vi "myRIO v1.0 Generate Register Values SPI.vi"(8 "error in (no error)":errorcluster, 11 "SPI Configuration v1.0":T1={"Frequency (Hz)"=0.0, "SPI Clock Phase"=enum."Leading", "SPI Clock Polarity"=enum."Low", "SPI Data Direction"=enum."Most significant bit first", "Frame Length"=1} {"Frame Length" min=1 max=16}) -> (0 "error out":errorcluster, 2 "SPI.CNFG":u16 format="%.0b", 3 "SPI.CNT":u16, 5 "Actual Frequency (Hz)":dbl)   [LabVIEW 2021]
uses:
  <vilib>/myRIO/Common/Instrument Driver Framework/myRIO v1.0/SPI/typedefs/SPI Configuration v1.0.ctl
  <vilib>/myRIO/Common/Instrument Driver Framework/myRIO v1.0/SPI/typedefs/SPI Clock Phase.ctl
  <vilib>/myRIO/Common/Instrument Driver Framework/myRIO v1.0/SPI/typedefs/SPI Clock Polarity.ctl
  <vilib>/myRIO/Common/Instrument Driver Framework/myRIO v1.0/SPI/typedefs/SPI Data Direction.ctl
  <vilib>/myRIO/Common/Instrument Driver Framework/myRIO v1.0/SPI/typedefs/SPI Frame Length.ctl
  <vilib>/myRIO/Common/Instrument Driver Framework/Utilities/typedefs/Clock Calculation Parameters.ctl
  <vilib>/myRIO/Common/Instrument Driver Framework/Utilities/vis/Calculate TOP (Phase Correct Mode).vi
  <vilib>/myRIO/Common/Instrument Driver Framework/Utilities/vis/Calculate TOP (Normal Mode).vi
  <vilib>/myRIO/Common/Instrument Driver Framework/Utilities/vis/Calculate Frequency (Phase Correct Mode).vi
  <vilib>/myRIO/Common/Instrument Driver Framework/Utilities/vis/Calculate Frequency (Normal Mode).vi
  <vilib>/Utility/error.llb/Error Cluster From Error Code.vi
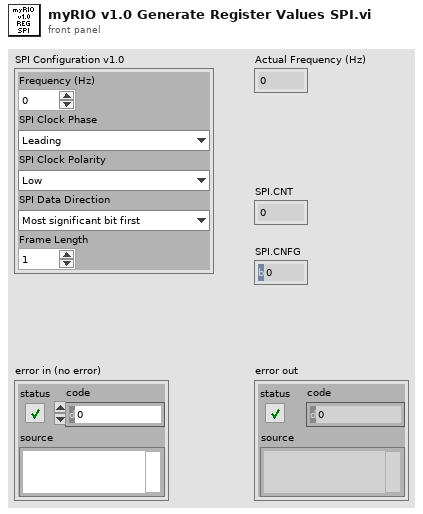
[diagram p1: front panel]
types:
  T1 = typedef "SPI Configuration v1.0.ctl" = cluster{"Frequency (Hz)":dbl, "SPI Clock Phase":T2, "SPI Clock Polarity":T3, "SPI Data Direction":T4, "Frame Length":T5}
  T2 = typedef "SPI Clock Phase.ctl" = enum8{"Leading", "Trailing"}
  T3 = typedef "SPI Clock Polarity.ctl" = enum8{"Low", "High"}
  T4 = typedef "SPI Data Direction.ctl" = enum8{"Most significant bit first", "Least significant bit first"}
  T5 = typedef "SPI Frame Length.ctl" = u8
  T6 = typedef "Clock Calculation Parameters.ctl" = cluster{"Base Clock Frequency (Hz)":dbl, "Max Counter Value":u32, "Min Counter Value":u32}
  T7 = typedef "Clock Settings.ctl" = cluster{"Clock Divisor":u32, "TOP":u32, "Actual Frequency (Hz)":dbl}
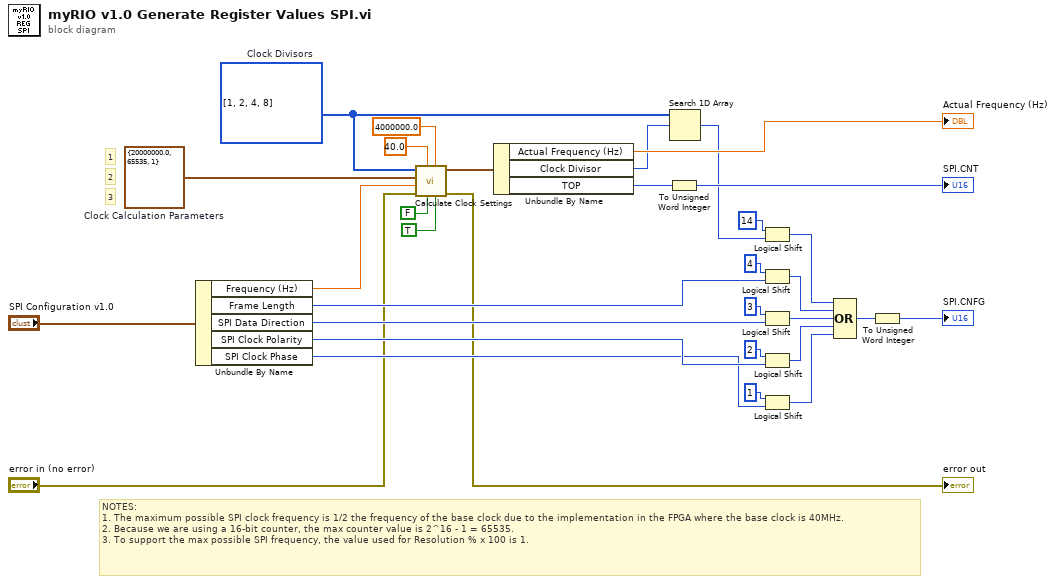
[diagram p0: block diagram]
diagram:
  w6 = T6 {"Base Clock Frequency (Hz)"=20000000.0, "Max Counter Value"=65535, "Min Counter Value"=1}  # Clock Calculation Parameters
  w7 = u32[] [1, 2, 4, 8]  # Clock Divisors
  # "3"
  # "2"
  # "1"
  # "NOTES:\n1. The maximum possible SPI clock frequency is 1/2 the frequency of the base clock due to the implementation in the FPGA where the base clock is 40MHz.\n2. Because we are using a 16-bit counter, the max counter value is 2^16 - 1 = 65535. \n3. To support the max possible SPI frequency, the value used for Resolution % x 100 is 1."
  n1 = Unbundle By Name("SPI Configuration v1.0") -> ("Frequency (Hz)"=w24:dbl, "Frame Length"=w28:T5, "SPI Data Direction"=w31:T4, "SPI Clock Polarity"=w30:T3, "SPI Clock Phase"=w29:T2)
  n2 = call <vilib>:"Calculate Clock Settings.vi"("Coerce Range?"=TRUE, "Max Frequency (Hz)"=4000000.0, "Phase Correct Mode?"=FALSE, "Min Frequency (Hz)"=40.0, "error in (no error)"="error in (no error)", "Requested Frequency (Hz)"=w24, "Clock Calculation Parameters"=w6, "Clock Divisors"=w7) -> ("error out"=→"error out":errorcluster, "Frequency Configuration"=w23:T7)  [unwired: 2 in]
  n3 = Unbundle By Name(w23) -> ("Actual Frequency (Hz)"=→"Actual Frequency (Hz)":dbl, "Clock Divisor"=w21:u32, "TOP"=w22:u32)
  n4 = To Unsigned Word Integer(number=w22) -> (unsigned 16bit integer=→"SPI.CNT":u16)
  n5 = Search 1D Array(1D array=w7, element=w21) -> (index of element=w9:i32)  [unwired: 1 in]
  n6 = Logical Shift(y=u16 14, x=w9) -> (x << y=w14:i32)
  n7 = Logical Shift(y=u16 4, x=w28) -> (x << y=w13:T5)
  n8 = Logical Shift(y=u16 3, x=w31) -> (x << y=w12:u32)
  n9 = Logical Shift(y=u16 2, x=w30) -> (x << y=w11:u32)
  n10 = Logical Shift(y=u16 1, x=w29) -> (x << y=w10:u32)
  n11 = Compound Arithmetic op=OR(w14, w13, w12, w11, w10) -> (w15:u32)
  n12 = To Unsigned Word Integer(number=w15) -> (unsigned 16bit integer=→"SPI.CNFG":u16)
